vi "Periodic Tasks.vi"(8 "error in":errorcluster) -> ()   [LabVIEW 2017]
doc: "This VI runs in parallel to other tasks. It can contain as many user-defined periodic loops as you need. These can carry out PID or other sorts of timed response."
uses:
  <vilib>/Rock Robotics/WPI/Utilities/WPI_GetSetVariantRefNum.vi
  Robot Global Data.vi
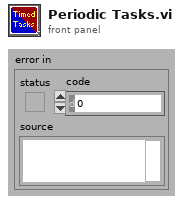
[diagram p1: front panel]
types:
  T1 = typedef "WPI_JoystickDevRef.ctl" = cluster{"Device":T2}
  T2 = typedef "WPI_JoystickDeviceEnum.ctl" = enum16{"USB 0", "USB 1", "USB 2", "USB 3", "USB 4", "USB 5"}
  T3 = typedef "WPI_RobotDriveDevRef.ctl" = cluster{"DevStatus":errorcluster, "Motors[]":T4[], "Square Inputs":bool, "Max Output":dbl}
  T4 = typedef "WPI_MotorControlDeviceRef.ctl" = cluster{"DeviceStatus":errorcluster, "Type":T5, "PWM":cluster{"PWM Channel":T6, "DeadBand":T7}, "CAN":cluster{"Device Number":u8, "SetOutput VI Ref":variant, "GetOutput VI Ref":variant, "Enable VI Ref":variant, "Disable VI Ref":variant, "Data":variant}, "Invert":bool, "DIO PWM":cluster{"PWM \"Enable\" Channel":T6, "DIOChannel":T8, "PWM Rate":dbl}}
  T5 = typedef "WPI_MotorControlType.ctl" = enum16{"PWM", "CAN", "DIO PWM"}
  T6 = typedef "FPGA_DIOPWMChannel.ctl" = enum8{"PWM 0", "PWM 1", "PWM 2", "PWM 3", "PWM 4", "PWM 5", "PWM 6", "PWM 7", "PWM 8", "PWM 9", "PWM MXP 0", "PWM MXP 1", "PWM MXP 2", "PWM MXP 3", "PWM MXP 4", "PWM MXP 5", "PWM MXP 6", "PWM MXP 7", "PWM MXP 8", "PWM MXP 9", "Invalid"}
  T7 = typedef "WPI_PWMDeadband.ctl" = cluster{"Name":string, "maxPositivePwm":i32, "minPositivePwm":i32, "centerPwm":i32, "maxNegativePwm":i32, "minNegativePwm":i32, "angularRange":u16}
  T8 = typedef "FPGA_DIOChannel.ctl" = enum8{"DIO 0", "DIO 1", "DIO 2", "DIO 3", "DIO 4", "DIO 5", "DIO 6", "DIO 7", "DIO 8", "DIO 9", "DIO MXP 0", "DIO MXP 1", "DIO MXP 2", "DIO MXP 3", "DIO MXP 4", "DIO MXP 5", "DIO MXP 6", "DIO MXP 7", "DIO MXP 8", "DIO MXP 9", "DIO MXP 10", "DIO MXP 11", "DIO MXP 12", "DIO MXP 13", "DIO MXP 14", "DIO MXP 15", "SPI Port CS1", "SPI Port CS2", "SPI Port CS3", "SPI Port MISO", "SPI Port MOSI", "Invalid"}
  T9 = cluster{"JoystickDevRef":T1, "RobotDriveDevRef":T3, "JoystickDevRef":T1, "JoystickDevRef":T1}
  T10 = typedef "WPI_EncoderDevRef.ctl" = cluster{"DevStatus":errorcluster, "EncoderIndex":T11, "CounterIndex":T12, "DistancePerCount":dbl, "Decoding Type":T13}
  T11 = typedef "FPGA_EncoderIdx.ctl" = enum8{"Enc 0", "Enc 1", "Enc 2", "Enc 3", "Enc 4", "Enc 5", "Enc 6", "Enc 7", "Invalid"}
  T12 = typedef "FPGA_CounterCtrSystemIndex.ctl" = enum8{"Ctr 0", "Ctr 1", "Ctr 2", "Ctr 3", "Ctr 4", "Ctr 5", "Ctr 6", "Ctr 7", "Invalid"}
  T13 = typedef "WPI_EncoderType.ctl" = enum16{"1x", "2x", "4x"}
  T14 = typedef "WPI_DigitalInputDevRef.ctl" = cluster{"DevStatus":errorcluster, "DIO Channel":T8}
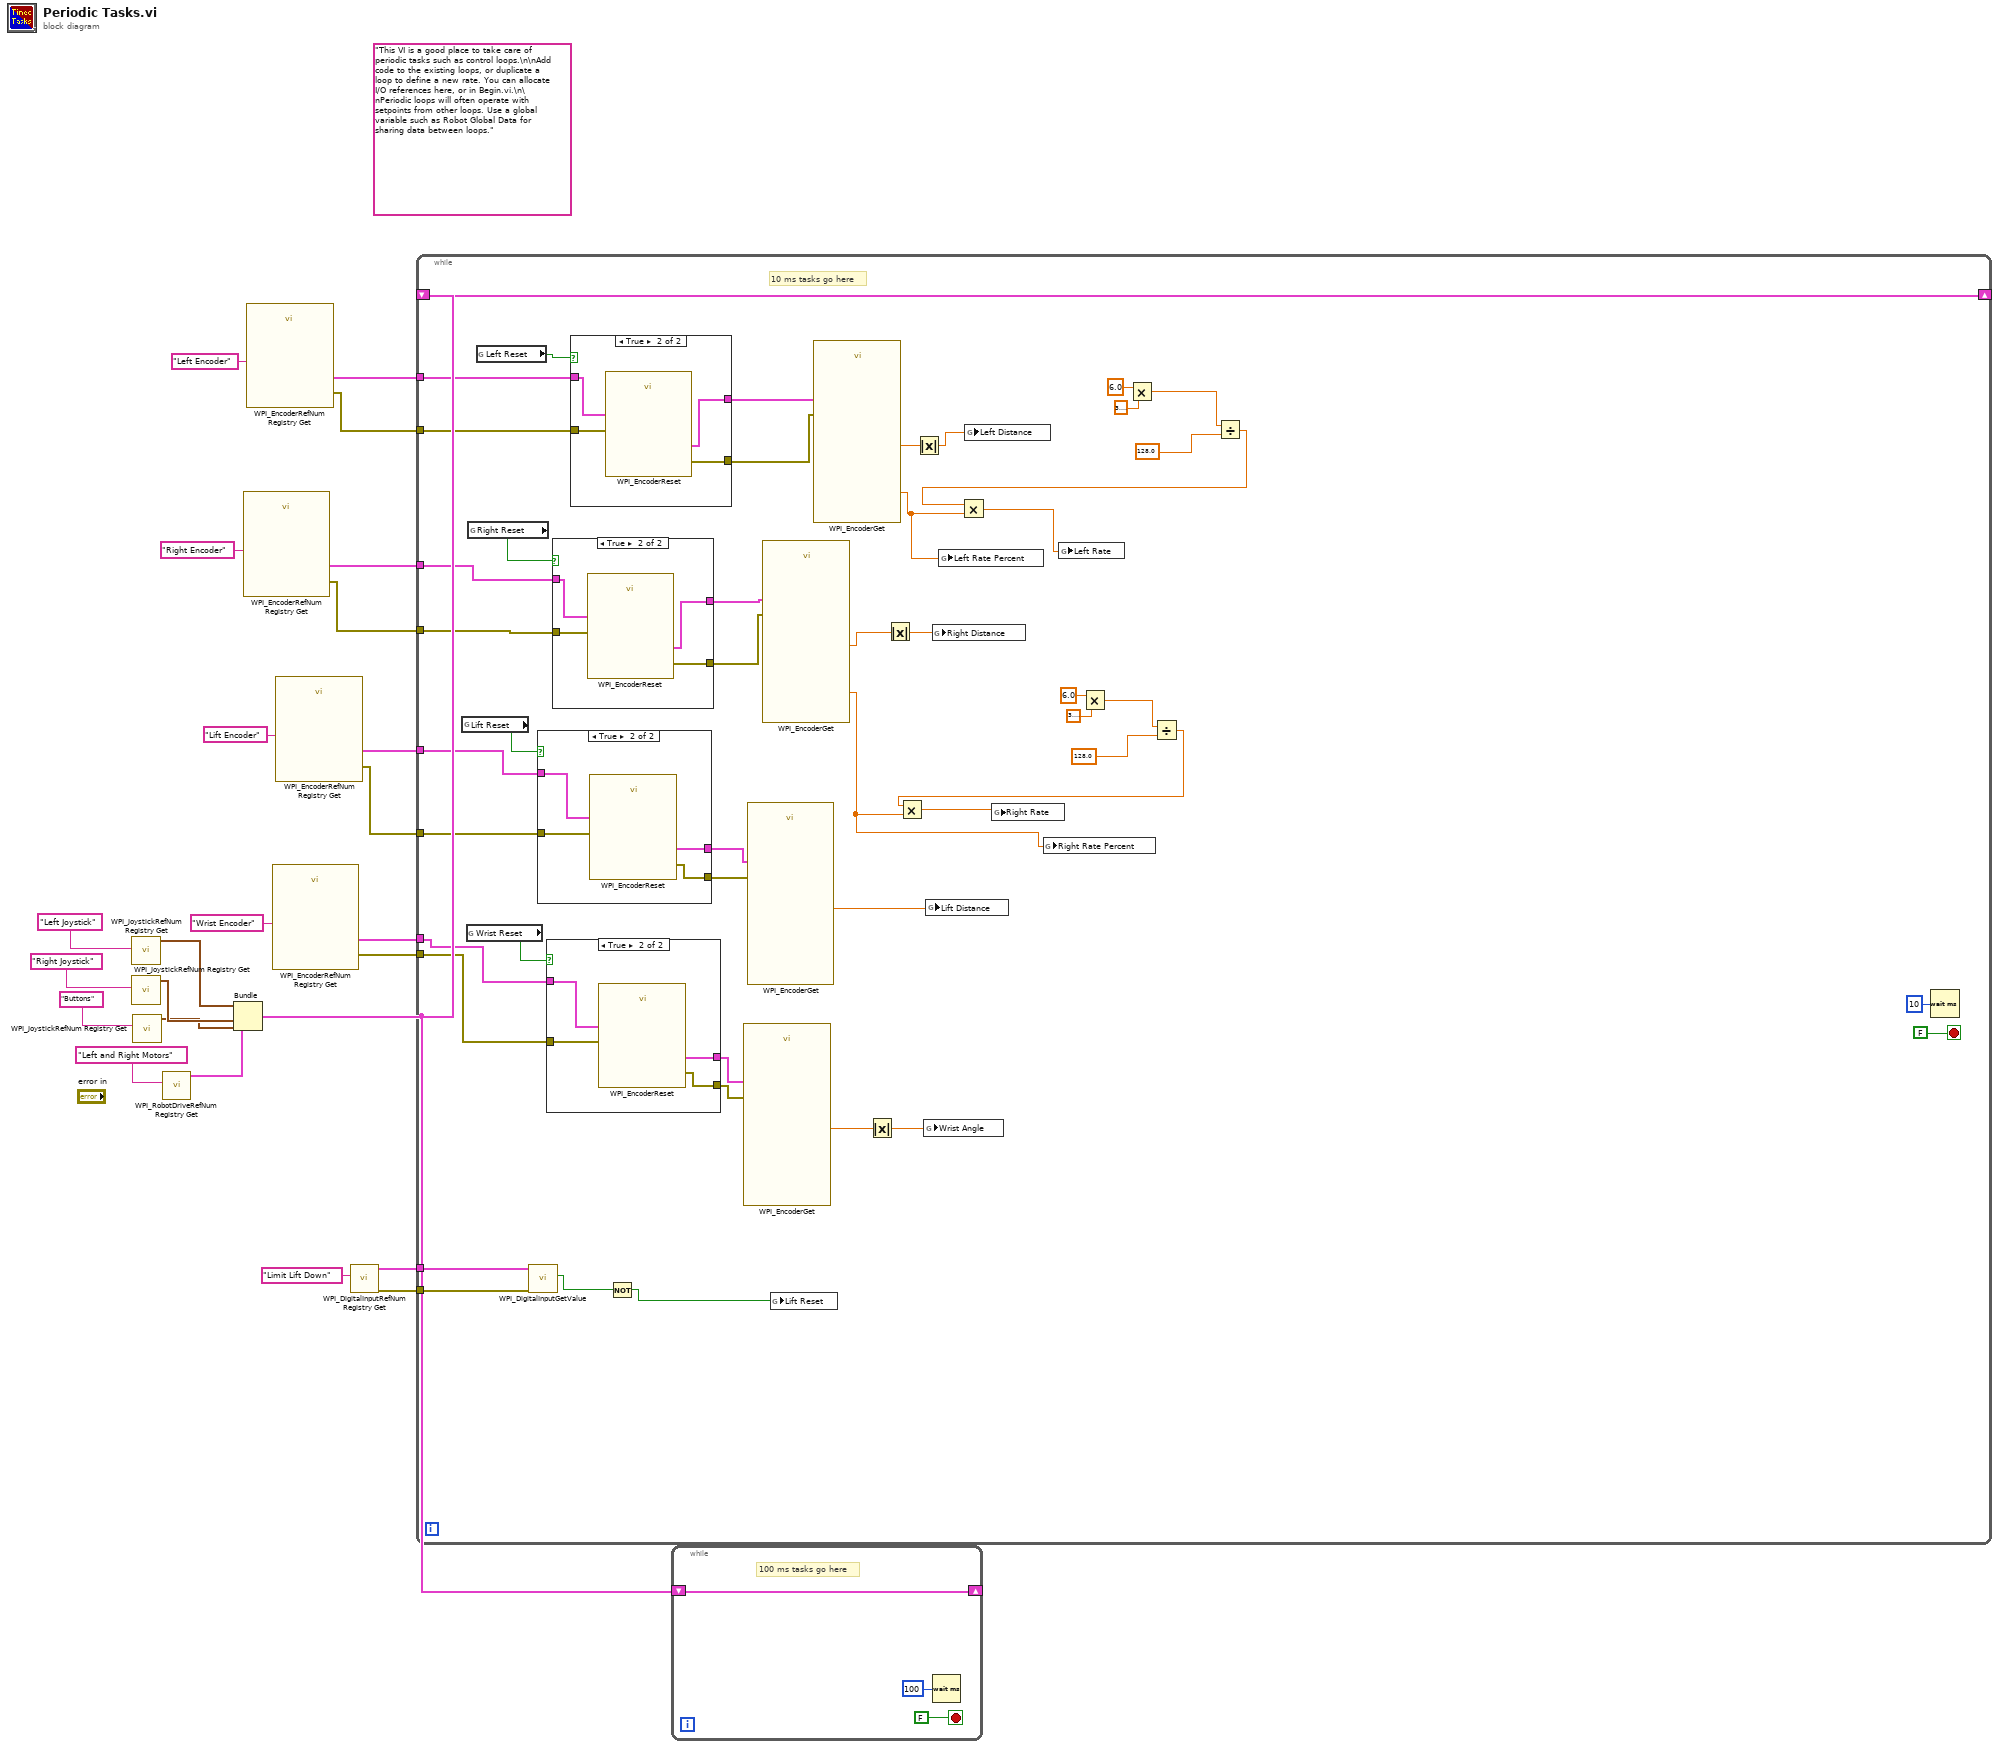
[diagram p0: block diagram]
diagram:
  (unwired) "This VI is a good place to take care of periodic tasks such as control loops.\n\nAdd code to the existing loops, or duplicate a loop to define a new rate. You can allocate I/O references here, or in Begin.vi.\n\nPeriodic loops will often operate with setpoints from other loops. Use a global variable such as Robot Global Data for sharing data between loops."
  n1 = call <vilib>:"WPI_JoystickRefNum Registry Get.vi"("refnum name"="Left Joystick") -> ("JoystickDevRef"=w22:T1)  [unwired: 1 in, 9 out]
  n2 = call <vilib>:"WPI_JoystickRefNum Registry Get.vi"("refnum name"="Right Joystick") -> ("JoystickDevRef"=w8:T1)  [unwired: 1 in, 9 out]
  n3 = call <vilib>:"WPI_JoystickRefNum Registry Get.vi"("refnum name"="Buttons") -> ("JoystickDevRef"=w7:T1)  [unwired: 1 in, 9 out]
  n4 = call <vilib>:"WPI_RobotDriveRefNum Registry Get.vi"("refnum name"="Left and Right Motors") -> ("RobotDriveDevRef"=w21:T3)  [unwired: 1 in, 9 out]
  n5 = Bundle("JoystickDevRef"=w22, "RobotDriveDevRef"=w21, "JoystickDevRef"=w8, "JoystickDevRef"=w7) -> (w20:T9)  [unwired: 1 out]
  n6 = call <vilib>:"WPI_EncoderRefNum Registry Get.vi"("refnum name"="Right Encoder") -> ("error out"=w14:errorcluster, "EncoderDevRef"=w16:T10)  [unwired: 9 in]
  n7 = call <vilib>:"WPI_EncoderRefNum Registry Get.vi"("refnum name"="Left Encoder") -> ("error out"=w15:errorcluster, "EncoderDevRef"=w17:T10)  [unwired: 9 in]
  n8 = call <vilib>:"WPI_EncoderRefNum Registry Get.vi"("refnum name"="Wrist Encoder") -> ("error out"=w4:errorcluster, "EncoderDevRef"=w11:T10)  [unwired: 9 in]
  n9 = call <vilib>:"WPI_EncoderRefNum Registry Get.vi"("refnum name"="Lift Encoder") -> ("error out"=w6:errorcluster, "EncoderDevRef"=w5:T10)  [unwired: 9 in]
  n10 = call <vilib>:"WPI_DigitalInputRefNum Registry Get.vi"("refnum name"="Limit Lift Down") -> ("error out"=w2:errorcluster, "DigitalInputDevRef"=w1:T14)  [unwired: 9 in]
  n11 = while {
    shift-right: [w70] -> _
    shift-left: w20 -> [w70]
    tunnel: w17 -> [w69]
    tunnel: w16 -> [w63]
    tunnel: w15 -> [w67]
    tunnel: w14 -> [w62]
    tunnel: w11 -> [w39]
    tunnel: w6 -> [w48]
    tunnel: w5 -> [w47]
    tunnel: w4 -> [w41]
    tunnel: w2 -> [w30]
    tunnel: w1 -> [w29]
    stop <- FALSE stop-if-true
    # "10 ms tasks go here"
    n12 = global read "Robot Global Data.vi" "Lift Reset"() -> (w44:bool)
    n13 = global read "Robot Global Data.vi" "Wrist Reset"() -> (w43:bool)
    n14 = global read "Robot Global Data.vi" "Right Reset"() -> (w61:bool)
    n15 = global read "Robot Global Data.vi" "Left Reset"() -> (w60:bool)
    n16 = call <vilib>:"WPI_DigitalInputGetValue.vi"("error in (no error)"=w30, "DigitalInputDevRef"=w29) -> ("Value"=w28:bool)  [unwired: 7 in, 2 out]
    n17 = case shown="True" w44 {
      tunnel: w48 -> [w79 w84]
      tunnel: w47 -> [w80 w83]
      tunnel: [w80 w82] -> w46
      tunnel: [w79 w81] -> w45
      frame False {
      }
      frame True {
        n18 = call <vilib>:"WPI_EncoderReset.vi"("error in (no error)"=w84, "EncoderDevRef"=w83) -> ("error out"=w81:errorcluster, "EncoderDevRef"=w82:T10)  [unwired: 8 in]
      }
    }
    n19 = case shown="True" w43 {
      tunnel: w41 -> [w73 w78]
      tunnel: w39 -> [w74 w77]
      tunnel: [w74 w76] -> w42
      tunnel: [w73 w75] -> w40
      frame False {
      }
      frame True {
        n20 = call <vilib>:"WPI_EncoderReset.vi"("error in (no error)"=w78, "EncoderDevRef"=w77) -> ("error out"=w75:errorcluster, "EncoderDevRef"=w76:T10)  [unwired: 8 in]
      }
    }
    n21 = case shown="True" w61 {
      tunnel: w63 -> [w86 w90]
      tunnel: [w86 w89] -> w65
      tunnel: w62 -> [w85 w88]
      tunnel: [w85 w87] -> w64
      frame False {
      }
      frame True {
        n22 = call <vilib>:"WPI_EncoderReset.vi"("error in (no error)"=w88, "EncoderDevRef"=w90) -> ("error out"=w87:errorcluster, "EncoderDevRef"=w89:T10)  [unwired: 8 in]
      }
    }
    n23 = case shown="True" w60 {
      tunnel: w69 -> [w92 w96]
      tunnel: [w92 w95] -> w68
      tunnel: w67 -> [w91 w94]
      tunnel: [w91 w93] -> w66
      frame False {
      }
      frame True {
        n24 = call <vilib>:"WPI_EncoderReset.vi"("error in (no error)"=w94, "EncoderDevRef"=w96) -> ("error out"=w93:errorcluster, "EncoderDevRef"=w95:T10)  [unwired: 8 in]
      }
    }
    n25 = Not(x=w28) -> (.not. x?=w27:bool)
    n26 = call <vilib>:"WPI_EncoderGet.vi"("error in (no error)"=w40, "EncoderDevRef"=w42) -> ("Distance"=w26:dbl)  [unwired: 4 in, 5 out]
    n27 = call <vilib>:"WPI_EncoderGet.vi"("error in (no error)"=w45, "EncoderDevRef"=w46) -> ("Distance"=w59:dbl)  [unwired: 4 in, 5 out]
    n28 = call <vilib>:"WPI_EncoderGet.vi"("error in (no error)"=w64, "EncoderDevRef"=w65) -> ("Distance"=w34:dbl, "Rate"=w36:dbl)  [unwired: 4 in, 4 out]
    n29 = global write "Robot Global Data.vi" "Lift Reset"(w27) -> ()
    n30 = call <vilib>:"WPI_EncoderGet.vi"("error in (no error)"=w66, "EncoderDevRef"=w68) -> ("Distance"=w32:dbl, "Rate"=w35:dbl)  [unwired: 4 in, 4 out]
    n31 = Absolute Value(x=w26) -> (abs(x)=w25:dbl)
    n32 = Absolute Value(x=w34) -> (abs(x)=w33:dbl)
    n33 = Absolute Value(x=w32) -> (abs(x)=w31:dbl)
    n34 = global write "Robot Global Data.vi" "Wrist Angle"(w25) -> ()
    n35 = global write "Robot Global Data.vi" "Lift Distance"(w59) -> ()
    n36 = global write "Robot Global Data.vi" "Right Distance"(w33) -> ()
    n37 = global write "Robot Global Data.vi" "Left Rate Percent"(w35) -> ()
    n38 = global write "Robot Global Data.vi" "Left Distance"(w31) -> ()
    n39 = global write "Robot Global Data.vi" "Right Rate Percent"(w36) -> ()
    n40 = Multiply(x=6.0, y=3.141592653589793) -> (x*y=w50:dbl)
    n41 = Multiply(x=6.0, y=3.141592653589793) -> (x*y=w49:dbl)
    n42 = Divide(x=w50, y=128.0) -> (x/y=w56:dbl)
    n43 = Multiply(x=w56, y=w36) -> (x*y=w55:dbl)
    n44 = global write "Robot Global Data.vi" "Right Rate"(w55) -> ()
    n45 = Divide(x=w49, y=128.0) -> (x/y=w51:dbl)
    n46 = Multiply(x=w51, y=w35) -> (x*y=w54:dbl)
    n47 = global write "Robot Global Data.vi" "Left Rate"(w54) -> ()
    n48 = Wait (ms)(milliseconds to wait=u32 10) -> ()  [unwired: 1 out]
  }
  n49 = while {
    shift-right: [w97] -> _
    shift-left: w20 -> [w97]
    stop <- FALSE stop-if-true
    # "100 ms tasks go here"
    n50 = Wait (ms)(milliseconds to wait=u32 100) -> ()  [unwired: 1 out]
  }
